vi "AddUSBLevel1TracePoint.vi"(8 "error in (no error)":errorcluster, 10 "trace log":string, 11 "Qbus in":refnum<class "Qbus.lvclass">) -> (0 "error out":errorcluster)   [LabVIEW 2017, in "USBDrive.lvlib"]
uses:
  <vilib>/addons/InsightCM/Devices/Shared/Common/USBDrive/USBDrive.lvlib
  <vilib>/addons/Qbus/Qbus.lvclass
  <vilib>/addons/TraceLogger/TraceLogger.lvlib
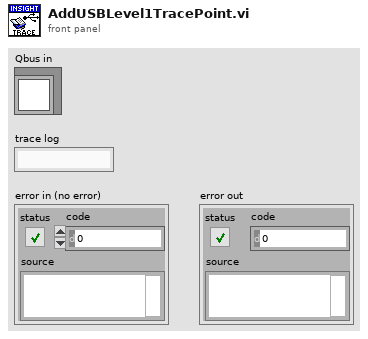
[diagram p1: front panel]
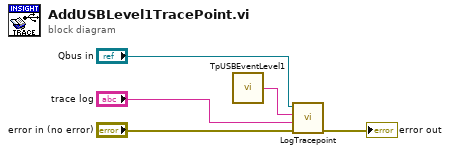
[diagram p0: block diagram]
diagram:
  n1 = call <vilib>:"TpUSBEventLevel1.vi"() -> ("TracepointName"=w1:string)  [unwired: 5 in]
  n2 = call <vilib>:"LogTracepoint.vi"("error in (no error)"="error in (no error)", "log string"="trace log", "tracepoint"=w1, "qbus in"="Qbus in") -> ("error out"=→"error out":errorcluster)  [unwired: 6 in, 1 out]
